vi "Counts to Angle.vi"(8 "Slope":dbl, 9 "y-intercept":dbl, 11 "Input Counts":dbl) -> (3 "Output Angle":dbl)   [LabVIEW 2013]
doc: "Conversion between counts and angle of the arm motor."
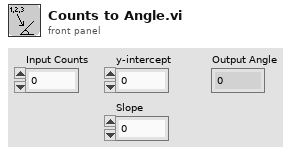
[diagram p1: front panel]
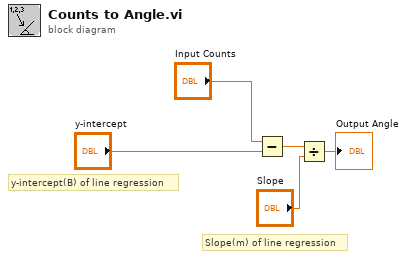
[diagram p0: block diagram]
diagram:
  # "Slope(m) of line regression"
  # "y-intercept(B) of line regression"
  n1 = Subtract(x="Input Counts", y="y-intercept") -> (x-y=w3:dbl)
  n2 = Divide(x=w3, y="Slope") -> (x/y=→"Output Angle":dbl)
